vi "Point in Rect.vi"(1 "point":cluster{"x":i16, "y":i16}, 2 "rect":T1) -> (0 "in rect?":bool)   [LabVIEW 2017]
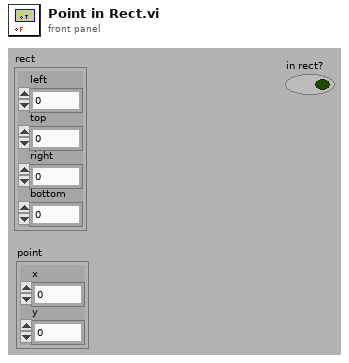
[diagram p1: front panel]
types:
  T1 = cluster{"left":i16, "top":i16, "right":i16, "bottom":i16}
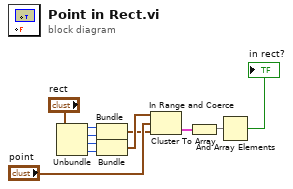
[diagram p0: block diagram]
diagram:
  n1 = Unbundle("rect") -> ("left"=w2:i16, "top"=w3:i16, "right"=w4:i16, "bottom"=w5:i16)
  n2 = Bundle("left"=w2, "top"=w3) -> (w6:cluster{"left":i16, "top":i16})  [unwired: 1 in]
  n3 = Bundle("right"=w4, "bottom"=w5) -> (w7:cluster{"right":i16, "bottom":i16})  [unwired: 1 in]
  n4 = In Range and Coerce(upper limit=w7, x="point", lower limit=w6) -> (In Range?=w9:cluster{"right":bool, "bottom":bool})  [unwired: 1 out]
  n5 = Cluster To Array(cluster=w9) -> (array=w10:bool[])
  n6 = And Array Elements(Boolean array=w10) -> (logical AND=→"in rect?":bool)
